vi "writeToXML.vi"(8 "error in (no error)":errorcluster, 10 "Class Label":string="TCSMccStatus", 11 "TCSMccStatus in":refnum<class "TCSMccStatus.lvclass">) -> (0 "error out":errorcluster, 2 "XML out":string="<>\n  <azElTracking>\n    <azimuthDemandedPosition>0</azimuthDemandedPosition>\n    <azVelocity>0</azVelocity>\n    <cableWrapDesired>C</cableWrapDesired>\n    <elevationDemandedPosition>0</elevationDemandedPosition>\n    <elVelocity>0</elVelocity>\n    <time>0</time>\n  </azElTracking>\n  <rotatorTracking>\n    <cableWrapDesired>C</cableWrapDesired>\n    <np>0</np>\n    <rotVelocity>0</rotVelocity>\n    <time>0</time>\n  </rotatorTracking>\n</>", 3 "TCSMccStatus out":refnum<class "TCSMccStatus.lvclass">)   [LabVIEW 2014, in "TCSDataDefinitions.lvlib" / "TCSMountControlStatus.lvlib" / "TCSMccStatus.lvclass"]
uses:
  TCSMccStatus.lvclass
  TCSMccStatus.lvclass/TCSMccStatus.ctl
  AzElTracking/AzElTracking/AzElTracking.lvclass
  RotatorTracking/RotatorTracking/RotatorTracking.lvclass
  <userlib>/Common/XML/XMLGenerator/XMLGenerator.lvclass
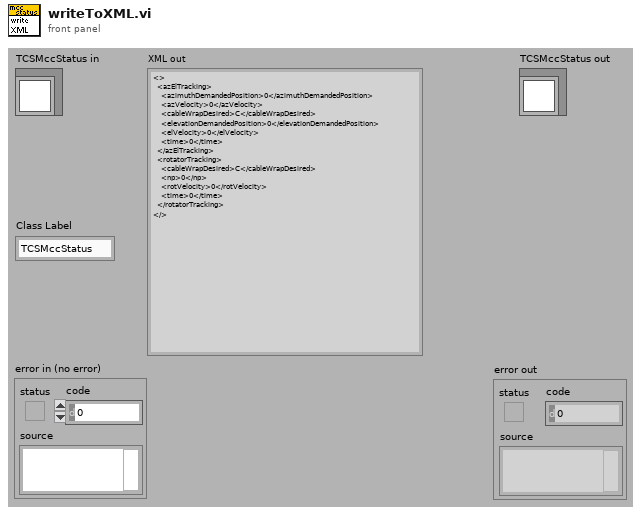
[diagram p1: front panel]
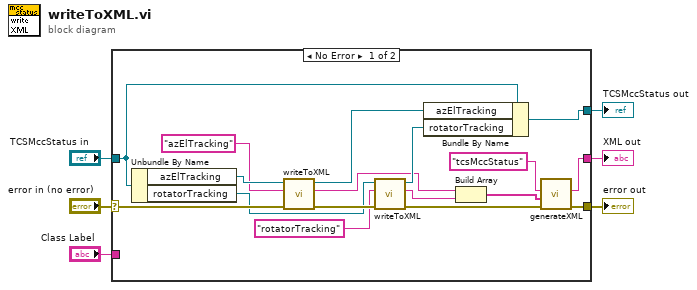
[diagram p0: block diagram]
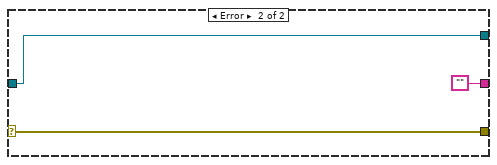
[diagram p2: hidden frame]
diagram:
  n1 = case shown="No Error" "error in (no error)" {
    selector: "error in (no error)" -> [w19 w26]
    tunnel: [w11 w26] -> w5
    tunnel: [w23 w25] -> w3
    tunnel: "TCSMccStatus in" -> [w22 w25]
    tunnel: [w10 ""] -> w2
    tunnel: "Class Label" -> [_ _]
    frame No Error {
      n2 = Unbundle By Name(w22) -> ("azElTracking"=w21:refnum<class "AzElTracking.lvclass">, "rotatorTracking"=w16:refnum<class "RotatorTracking.lvclass">)
      n3 = call-dynamic "writeToXML.vi"("error in (no error)"=w19, "Class Label"="azElTracking", "AzElTracking in"=w21) -> ("error out"=w18:errorcluster, "XML out"=w15:string, "AzElTracking out"=w20:refnum<class "AzElTracking.lvclass">)  [unwired: 6 in]
      n4 = call-dynamic "writeToXML.vi"("error in (no error)"=w18, "Class Label"="rotatorTracking", "RotatorTracking in"=w16) -> ("error out"=w12:errorcluster, "XML out"=w14:string, "RotatorTracking out"=w17:refnum<class "RotatorTracking.lvclass">)  [unwired: 6 in]
      n5 = Bundle By Name(cluster=w22, "azElTracking"=w20, "rotatorTracking"=w17) -> (w23:refnum<class "TCSMccStatus.lvclass">)
      n6 = Build Array(w15, w14) -> (w13:string[])
      n7 = call <userlib>:"generateXML.vi"("error in"=w12, "childrenXML"=w13, "elementName"="tcsMccStatus" ("Class Label")) -> ("error out"=w11:errorcluster, "XML out"=w10:string)  [unwired: 6 in, 1 out]
    }
    frame Error {
    }
  }
  "error out" <- w5
  "TCSMccStatus out" <- w3
  "XML out" <- w2
